vi "IS Process Response.vi"(8 "Error In (no error)":errorcluster, 10 "Response Body":string, 11 "Response Headers":string) -> (0 "Error Out":errorcluster, 3 "Rate Limit Reached":bool)   [LabVIEW 2013]
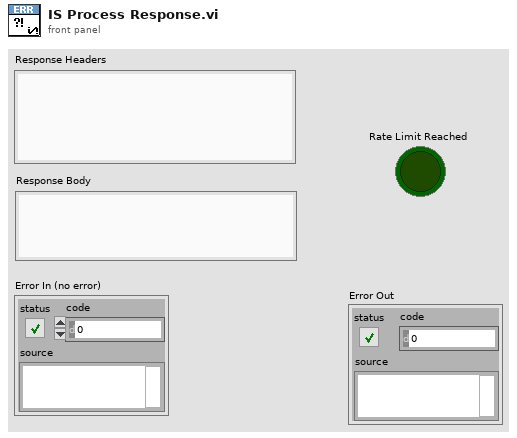
[diagram p1: front panel]
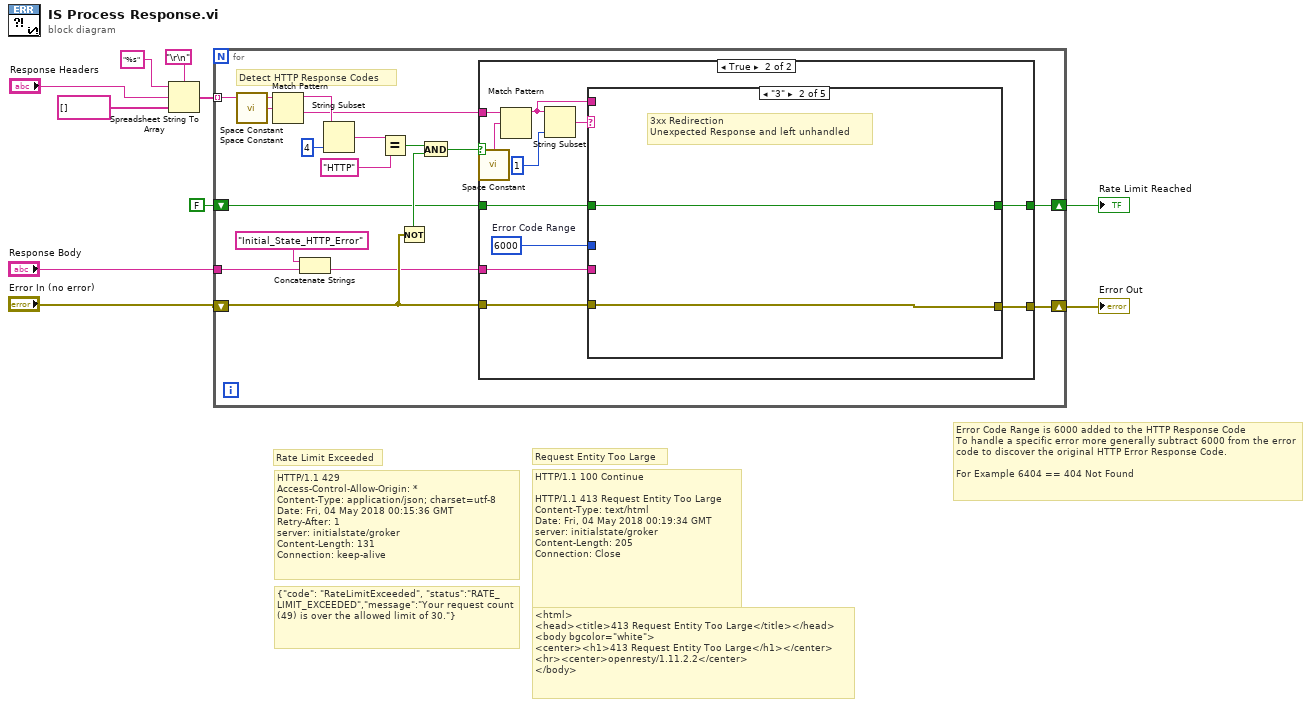
[diagram p0: block diagram]
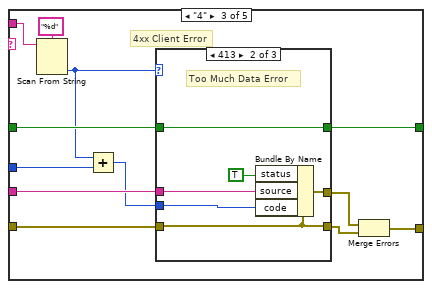
[diagram p4: hidden frame]
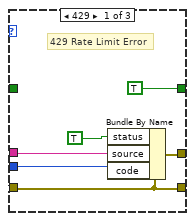
[diagram p5: hidden frame]
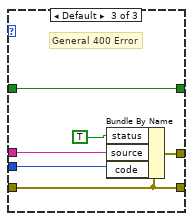
[diagram p6: hidden frame]
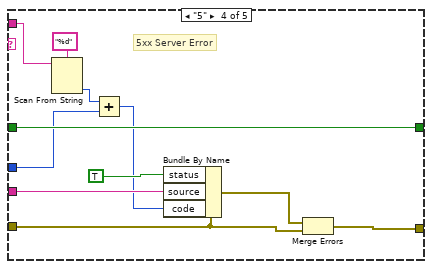
[diagram p7: hidden frame]
diagram:
  # "Error Code Range is 6000 added to the HTTP Response Code\nTo handle a specific error more generally subtract 6000 from the error code to discover the original HTTP Error Response Code. \n\nFor Example 6404 == 404 Not Found"
  # "<html>\n<head><title>413 Request Entity Too Large</title></head>\n<body bgcolor=\"white\">\n<center><h1>413 Request Entity Too Large</h1></center>\n<hr><center>openresty/1.11.2.2</center>\n</body>"
  # "Request Entity Too Large"
  # "HTTP/1.1 100 Continue\n\nHTTP/1.1 413 Request Entity Too Large\nContent-Type: text/html\nDate: Fri, 04 May 2018 00:19:34 GMT\nserver: initialstate/groker\nContent-Length: 205\nConnection: Close"
  # "{\"code\": \"RateLimitExceeded\", \"status\":\"RATE_LIMIT_EXCEEDED\",\"message\":\"Your request count (49) is over the allowed limit of 30.\"}"
  # "Rate Limit Exceeded"
  # "HTTP/1.1 429 \nAccess-Control-Allow-Origin: *\nContent-Type: application/json; charset=utf-8\nDate: Fri, 04 May 2018 00:15:36 GMT\nRetry-After: 1\nserver: initialstate/groker\nContent-Length: 131\nConnection: keep-alive"
  n1 = Spreadsheet String To Array(delimiter (Tab)="\r\n", format string="%s", spreadsheet string="Response Headers", array type (2D Dbl)=string[] []) -> (array=w6:string[])
  n2 = for {
    tunnel: w6 -> [w27] mode=indexing
    tunnel: "Response Body" -> [w13]
    shift-right: [w20] -> w3
    shift-left: "Error In (no error)" -> [w17]
    shift-right: [w15] -> w1
    shift-left: FALSE -> [w14]
    # "Detect HTTP Response Codes"
    n3 = call <vilib>:"Space Constant.vi"() -> ()  [unwired: 1 out]
    n4 = call <vilib>:"Space Constant.vi"() -> ("String"=w26:string)
    n5 = Match Pattern(string=w27, regular expression=w26) -> (before substring=w25:string, after substring=w21:string)  [unwired: 1 in, 2 out]
    n6 = Concatenate Strings("Initial_State_HTTP_Error", w13) -> (w12:string)
    n7 = String Subset(string=w25, length (rest)=4 ("length (rest)")) -> (substring=w23:string)  [unwired: 1 in]
    n8 = Equal?(x=w23, y="HTTP") -> (x = y?=w19:bool)
    n9 = Not(x=w17) -> (.not. x?=w18:bool)
    n10 = And(x=w19, y=w18) -> (x .and. y?=w16:bool)
    n11 = case shown="True" w16 {
      tunnel: w21 -> [_ w40]
      tunnel: w17 -> [w29 w36]
      tunnel: w12 -> [_ w35]
      tunnel: [w29 w30] -> w20
      tunnel: [w28 w34] -> w15
      tunnel: w14 -> [w28 w33]
      frame False {
      }
      frame True {
        w32 = 6000  # Error Code Range
        n12 = call <vilib>:"Space Constant.vi"() -> ("String"=w39:string)
        n13 = Match Pattern(string=w40, regular expression=w39) -> (before substring=w31:string)  [unwired: 1 in, 3 out]
        n14 = String Subset(string=w31, length (rest)=1 ("length (rest)")) -> (substring=w37:string)  [unwired: 1 in]
        n15 = case shown="\"3\"" w37 {
          tunnel: w36 -> [w41 w43 w56 w76 w86]
          tunnel: w35 -> [_ _ w55 w85 _]
          tunnel: [w42 w44 w54 w83 w87] -> w34
          tunnel: w33 -> [w42 w44 w53 w83 w87]
          tunnel: w32 -> [_ _ w51 w80 _]
          tunnel: w31 -> [_ _ w48 w78 _]
          tunnel: [w41 w43 w45 w75 w86] -> w30
          frame "2" {
            # "2xx Response Codes\nEverything OK Ignore"
          }
          frame "3" {
            # "3xx Redirection\nUnexpected Response and left unhandled"
          }
          frame "4" {
            # "4xx Client Error"
            n16 = Scan From String(format string="%d", input string=w48) -> (output 1=w49:i32)  [unwired: 3 in, 3 out]
            n17 = Add(x=w49, y=w51) -> (x+y=w50:i32)
            n18 = case shown="413" w49 {
              tunnel: w56 -> [w57 w63 w69]
              tunnel: w55 -> [w61 w67 w73]
              tunnel: [w60 w66 w72] -> w47
              tunnel: [TRUE w65 w71] -> w54
              tunnel: w53 -> [_ w65 w71]
              tunnel: w50 -> [w58 w64 w70]
              tunnel: [w57 w63 w69] -> w46
              frame 429 {
                # "429 Rate Limit Error"
                n19 = Bundle By Name(cluster=w57, "status"=TRUE, "source"=w61, "code"=w58) -> (w60:errorcluster)
              }
              frame 413 {
                # "Too Much Data Error"
                n20 = Bundle By Name(cluster=w63, "status"=TRUE, "source"=w67, "code"=w64) -> (w66:errorcluster)
              }
              frame Default {
                # "General 400 Error"
                n21 = Bundle By Name(cluster=w69, "status"=TRUE, "source"=w73, "code"=w70) -> (w72:errorcluster)
              }
            }
            n22 = Merge Errors(w47, w46) -> (w45:errorcluster)
          }
          frame "5" {
            # "5xx Server Error"
            n23 = Scan From String(format string="%d", input string=w78) -> (output 1=w81:i32)  [unwired: 3 in, 3 out]
            n24 = Add(x=w81, y=w80) -> (x+y=w79:i32)
            n25 = Bundle By Name(cluster=w76, "status"=TRUE, "source"=w85, "code"=w79) -> (w77:errorcluster)
            n26 = Merge Errors(w77, w76) -> (w75:errorcluster)
          }
          frame "1", Default {
            # "1xx Response \nIgnore"
          }
        }
      }
    }
  }
  "Error Out" <- w3
  "Rate Limit Reached" <- w1
